vi "Not a Valid UI.vi"(1 "Flex UI in":refnum<class "Flex UI.lvclass">) -> (0 "Not a Valid UI":bool)   [LabVIEW 2016, in "Flex UI.lvclass"]
uses:
  Flex UI.lvclass
  Flex UI.lvclass/Flex UI.ctl
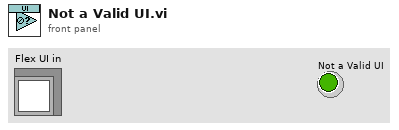
[diagram p1: front panel]
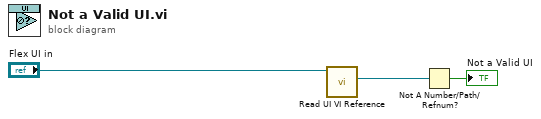
[diagram p0: block diagram]
diagram:
  n1 = call "Read UI VI Reference.vi"("Flex UI in"="Flex UI in") -> ("UI VI Reference"=w2:refnum<vi>)  [unwired: 9 in, 1 out]
  n2 = Not A Number/Path/Refnum?(number/path/refnum=w2) -> (NaN/Path/Refnum?=→"Not a Valid UI":bool)
